vi "getCircle.vi"(8 "error in (no error)":errorcluster, 10 "color":string, 11 "fwShapeFactory in":refnum<class "fwShapeFactory.lvclass">) -> (0 "error out":errorcluster, 2 "fwCircle.lvclass":refnum<class "fwCircle.lvclass">, 3 "fwShapeFactory out":refnum<class "fwShapeFactory.lvclass">)   [LabVIEW 2017, in "fwShapeFactory.lvclass"]
uses:
  fwShapeFactory.lvclass
  Circle Class/fwCircle.lvclass
  C:/Users/fflores/Documents/LabVIEW-Open-Projects/LabIVEW OOP Design Patterns/Flightweight Pattern/Shape Class/fwShape.lvclass
  fwShapeFactory.lvclass/fwShapeFactory.ctl
  ConsoleOut/Print Options.ctl
  Circle Class/fwCircle.lvclass/fwCircle.ctl
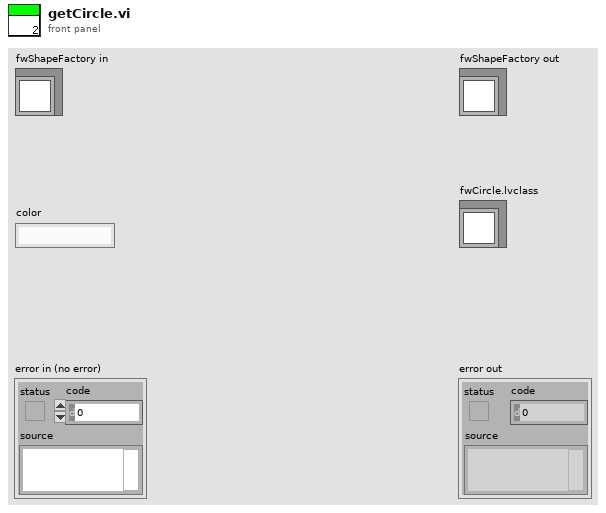
[diagram p1: front panel]
types:
  T1 = typedef "Print Options.ctl" = enum16{"Create", "Get Reference", "Print", "Print Header", "Close"}
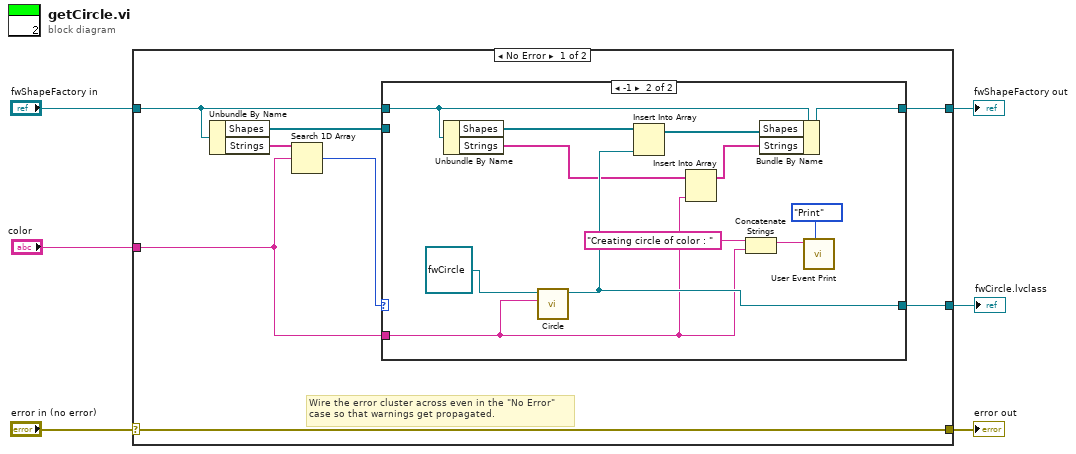
[diagram p0: block diagram]
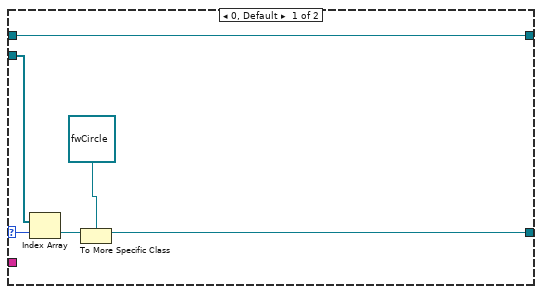
[diagram p2: hidden frame]
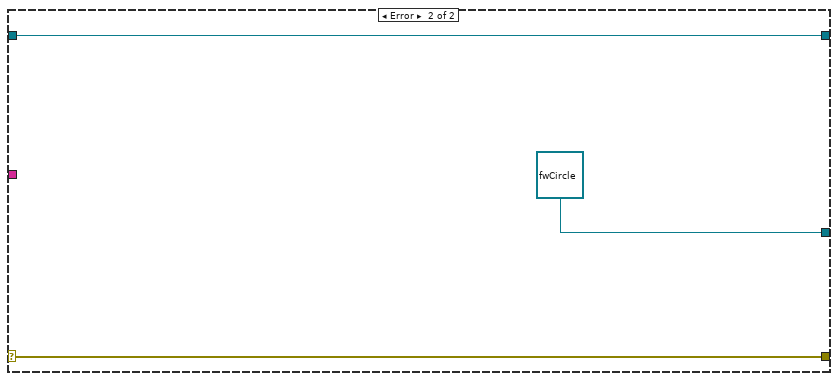
[diagram p3: hidden frame]
diagram:
  n1 = case shown="No Error" "error in (no error)" {
    selector: "error in (no error)" -> [w14 w35]
    tunnel: [w14 w35] -> w5
    tunnel: [w8 w34] -> w3
    tunnel: "fwShapeFactory in" -> [w9 w34]
    tunnel: "color" -> [w7 _]
    tunnel: [w11 refnum<class "fwCircle.lvclass"> refnum ("fwCircle.lvclass")] -> w1
    frame No Error {
      # "Wire the error cluster across even in the \"No Error\"\ncase so that warnings get propagated."
      n2 = Unbundle By Name(w9) -> ("Shapes"=w12:refnum<class "fwShape.lvclass">[], "Strings"=w13:string[])
      n3 = Search 1D Array(1D array=w13, element=w7) -> (index of element=w10:i32)  [unwired: 1 in]
      n4 = case shown="-1" w10 {
        selector: w10 -> [w16 _]
        tunnel: w12 -> [w20 _]
        tunnel: [w18 w27] -> w11
        tunnel: [w15 w31] -> w8
        tunnel: w9 -> [w15 w30]
        tunnel: w7 -> [_ w23]
        frame 0, Default {
          n5 = Index Array(array=w20, index=w16) -> (element=w19:refnum<class "fwShape.lvclass">)
          n6 = To More Specific Class(target class=refnum<class "fwCircle.lvclass"> refnum ("fwCircle.lvclass"), reference=w19) -> (specific class reference=w18:refnum<class "fwCircle.lvclass">)  [unwired: 1 in, 1 out]
        }
        frame -1 {
          n7 = Unbundle By Name(w30) -> ("Shapes"=w29:refnum<class "fwShape.lvclass">[], "Strings"=w24:string[])
          n8 = call "Circle.vi"("color"=w23, "fwCircle in"=refnum<class "fwCircle.lvclass"> refnum ("fwCircle.lvclass")) -> ("fwCircle out"=w27:refnum<class "fwCircle.lvclass">)  [unwired: 8 in, 1 out]
          n9 = Insert Into Array(array=w29, new element=w27) -> (w28:refnum<class "fwShape.lvclass">[])  [unwired: 1 in]
          n10 = Insert Into Array(array=w24, new element=w23) -> (w25:string[])  [unwired: 1 in]
          n11 = Concatenate Strings("Creating circle of color : " ("message"), w23) -> (w22:string)
          n12 = Bundle By Name(cluster=w30, "Shapes"=w28, "Strings"=w25) -> (w31:refnum<class "fwShapeFactory.lvclass">)
          n13 = call "User Event Print.vi"("Options"=Print_Options."Print", "String to Print"=w22) -> ()  [unwired: 8 in, 2 out]
        }
      }
    }
    frame Error {
    }
  }
  "error out" <- w5
  "fwShapeFactory out" <- w3
  "fwCircle.lvclass" <- w1
